vi "Affiche Message operateur.vi"(8 "error in (no error)":errorcluster caption="entrée d'erreur (pas d'erreur)", 9 "Etat en cours":string, 10 "Fonction Appelante":T1=enum."End", 11 "Afficher ?":bool) -> (0 "error out":errorcluster caption="sortie d'erreur")   [LabVIEW 2020]
uses:
  TypeDef/Liste Fonction appelante.ctl
  Type DEF/Commande Event Demande Op.ctl
  IHM/Variable globale.vi
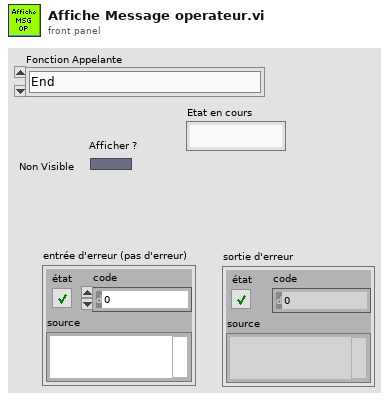
[diagram p1: front panel]
types:
  T1 = typedef "Liste Fonction appelante.ctl" = enum16{"None", "Open Com DUT", "Enter OF", "Serial Number", "Start-up", "Start Test", "Finish", "Enter S/N PWR", "Enter S/N ANT", "Read Mac Address", "Test Frequency", "Initialization", "ID EnOcean", "ID Wirepass", "Test Button", "Test EEPROM", "Test LED", "Test Relay", "Test RTC", "Reset Factory", "Read parameter", "Programm Software", "Programm FW", "IHM", "Print Label PCBA", "Print Label Assembled", "Print Label Packaging", "End", "Error"}
  T2 = typedef "Commande Event Demande Op.ctl" = cluster{"Action":enum16{"None", "Quit", "Hidden", "Visible", "Affiche bouton", "Masque bouton"}, "Fonction Appelante":T1, "Nom etape":string, "error in (no error)":errorcluster}
  T3 = typedef "File et notification.ctl" = cluster{"Arret Appli":refnum<notifier>, "Erreur Acqui":refnum<notifier>, "File Event Sequenceur":refnum<queue>, "Liste test à faire":refnum<queue>, "File Event Historique":refnum<queue>, "Variable Global":refnum<notifier>, "Variable stocke retour Etat":refnum<notifier>, "Retour Validation OP":refnum<queue>, "Demande Validation OP":refnum<queue>, "Retour Autotest":refnum<notifier>, "Demande Autotest":refnum<queue>, "Adr Mac Produit":refnum<notifier>, "Autorise commande":refnum<notifier>, "Event Init BLE":refnum<notifier>, "Action Lecture RS":refnum<queue>, "Key produit":refnum<notifier>, "Retour Saisie OP":refnum<queue>, "Demande Saisie OP":refnum<queue>, "Etat flashage":refnum<notifier>, "Code Operateur":refnum<notifier>, "Resultat test Global":refnum<notifier>, "Stop Test":refnum<notifier>, "Init IHM Autotest":refnum<notifier>, "Version test bench":refnum<notifier>, "SN Product":refnum<notifier>, "En erreur":refnum<notifier>, "Affiche Result":refnum<queue>, "S/N PWR":refnum<notifier>, "AppEUI":refnum<notifier>, "Action Lecture Temp":refnum<queue>, "Temp":refnum<notifier>, "AppKey":refnum<notifier>, "OF":refnum<notifier>, "File Commande Shielding":refnum<queue>, "Return Status":refnum<notifier>, "ID Product":refnum<notifier>, "Version FW":refnum<notifier>, "Version HW":refnum<notifier>, "Adresse IHM":refnum<notifier>, "RTC":refnum<notifier>, "S/N Ant":refnum<notifier>, "SN Encode":refnum<notifier>, "Key Product":refnum<notifier>}
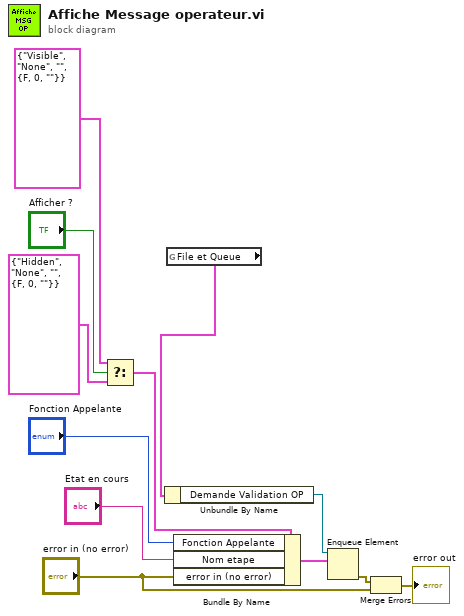
[diagram p0: block diagram]
diagram:
  n1 = Select(t=T2 {"Action"=enum."Visible", "Fonction Appelante"=enum."None", "Nom etape"="", "error in (no error)"={"status"=FALSE, "code"=0, "source"=""}} ("élément"), s="Afficher ?", f=T2 {"Action"=enum."Hidden", "Fonction Appelante"=enum."None", "Nom etape"="", "error in (no error)"={"status"=FALSE, "code"=0, "source"=""}} ("élément")) -> (s? t:f=w9:T2)
  n2 = global read "Variable globale.vi" "File et Queue"() -> (w1:T3)
  n3 = Unbundle By Name(w1) -> ("Demande Validation OP"=w5:refnum<queue>)
  n4 = Bundle By Name(cluster=w9, "Fonction Appelante"="Fonction Appelante", "Nom etape"="Etat en cours", "error in (no error)"="error in (no error)") -> (w8:T2)
  n5 = Enqueue Element(queue=w5, element=w8) -> (error out=w7:errorcluster)  [unwired: 2 in, 2 out]
  n6 = Merge Errors(w7, "error in (no error)") -> (→"error out":errorcluster)
